vi "test_Byte coerced response.vi"(8 "error in (no error)":errorcluster, 11 "TestCase in":refnum<class "Instrument Addon Host API Tests.lvclass">) -> (0 "error out":errorcluster, 3 "TestCase out":refnum<class "Instrument Addon Host API Tests.lvclass">)   [LabVIEW 2019, in "Instrument Addon Host API Tests.lvclass"]
uses:
  Instrument Addon Host API Tests.lvclass
  Addon/Addon Shared/Types/Buffered RT Instrument Command.ctl
  Addon/Addon Shared/Types/Response Wait Type.ctl
  <vilib>/addons/_JKI Toolkits/VI Tester/TestCase.llb/TestCase.lvclass
  APIs/Host Automation API/Instrument Host Automation API.lvlib
  Addon/Addon Shared/Instrument Addon Shared.lvlib
  C:/Program Files (x86)/National Instruments/LabVIEW 2019/vi.lib/addons/_JKI Toolkits/VI Tester/TestCase.llb/TestCase.lvclass
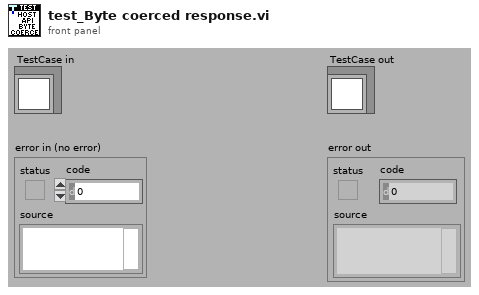
[diagram p1: front panel]
types:
  T1 = typedef "Instrument Addon Shared.lvlib/Buffered RT Instrument Command.ctl" = cluster{"Command":string, "Response Expected?":bool, "Wait Type":T2, "Wait Value":dbl}
  T2 = typedef "Instrument Addon Shared.lvlib/Response Wait Type.ctl" = enum16{"Byte Count", "Wait sec"}
  T3 = typedef "NI STM.lvlib/TCP Connection Info.ctl" = cluster{"connection ID":refnum<k5>, "meta data":T4[]}
  T4 = typedef "NI STM.lvlib/MetaDataElement.ctl" = string
  T5 = typedef "Instrument Addon Shared.lvlib/Buffered RT Instrument Request.ctl" = cluster{"Response":string, "Error":errorcluster}
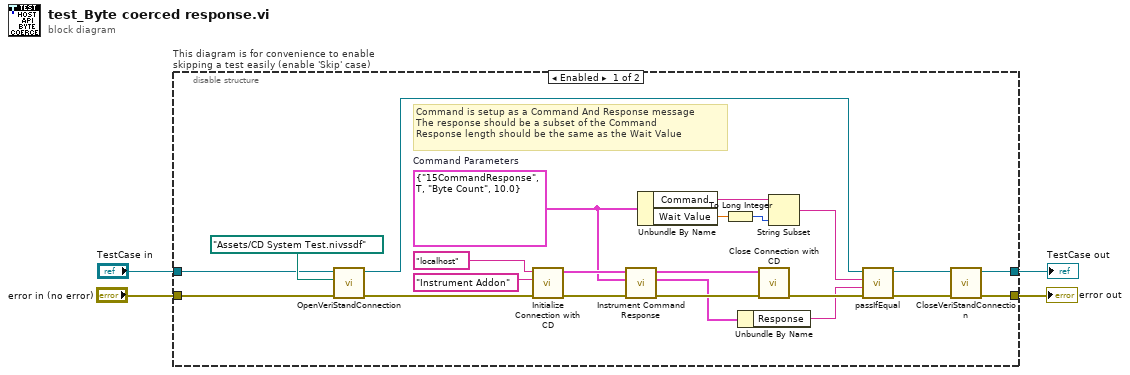
[diagram p0: block diagram]
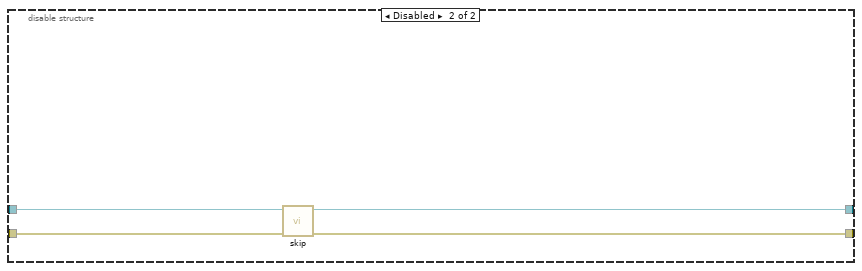
[diagram p2: hidden frame]
diagram:
  n1 = disable-structure "This diagram is for convenience to enable skipping a test easily (enable 'Skip' case)" shown="Enabled" {
    disable-tunnel: "TestCase in" -> [w23 w31]
    disable-tunnel: [w21 w29] -> w1
    disable-tunnel: [w22 w30] -> w3
    disable-tunnel: "error in (no error)" -> [w24 w28]
    frame Enabled {
      w11 = T1 {"Command"="15CommandResponse", "Response Expected?"=TRUE, "Wait Type"=enum."Byte Count", "Wait Value"=10.0}  # Command Parameters
      # "Command is setup as a Command And Response message\nThe response should be a subset of the Command\nResponse length should be the same as the Wait Value"
      n2 = call-dynamic "OpenVeriStandConnection.vi"("error in (no error)"=w24, "System Definition File"=path "Assets/CD System Test.nivssdf", "VeriStand Test Case in"=w23) -> ("error out"=w20:errorcluster, "VeriStand Test Case out"=w13:refnum<class "Instrument Addon Host API Tests.lvclass">)  [unwired: 6 in, 1 out]
      n3 = call "Initialize Connection with CD.vi"("error in (no error)"=w20, "TCP Service"="Instrument Addon", "IP Address"="localhost") -> ("error out"=w17:errorcluster, "connection info out"=w12:T3)  [unwired: 7 in]
      n4 = call "Instrument Command Response.vi"("error in (no error)"=w17, "Command Parameters"=w11, "Comm.Info"=w12) -> ("error out"=w15:errorcluster, "Response"=w10:T5, "Comm.Info"=w14:T3)  [unwired: 5 in, 1 out]
      n5 = Unbundle By Name(w11) -> ("Command"=w8:string, "Wait Value"=w6:dbl)
      n6 = To Long Integer(number=w6) -> (32bit integer=w5:i32)
      n7 = Unbundle By Name(w10) -> ("Response"=w9:string)
      n8 = call "Close Connection with CD.vi"("error in"=w15, "Comm.Info"=w14) -> ("error out"=w16:errorcluster)  [unwired: 9 in]
      n9 = String Subset(string=w8, length (rest)=w5) -> (substring=w7:string)  [unwired: 1 in]
      n10 = call-dynamic "passIfEqual.vi"("error in (no error)"=w16, "y"=w9, "x"=w7, "TestCase in"=w13) -> ("error out"=w19:errorcluster, "TestCase out"=w18:refnum<class "Instrument Addon Host API Tests.lvclass">)  [unwired: 6 in]
      n11 = call-dynamic "CloseVeriStandConnection.vi"("error in (no error)"=w19, "VeriStand Test Case in"=w18) -> ("error out"=w22:errorcluster, "VeriStand Test Case out"=w21:refnum<class "Instrument Addon Host API Tests.lvclass">)  [unwired: 8 in]
    }
    frame Disabled {
      # "skip test result while test is under development"
      n12 = call <vilib>:"skip.vi"("error in (no error)"=w28, "TestCase in"=w31) -> ("error out"=w30:errorcluster, "TestCase out"=w29:refnum<class "Instrument Addon Host API Tests.lvclass">)  [unwired: 8 in]
    }
  }
  "error out" <- w3
  "TestCase out" <- w1
